vi "GetImage.vi"(8 "error in (no error)":errorcluster, 10 "index (0 = most recent)":i32) -> (0 "error out":errorcluster, 2 "Img":string)   [LabVIEW 2017, in "SystemController.lvclass"]
doc: "---------------------------------------------------------------\nJKI State Machine Objects™\nhttp://jki.net/state-machine-objects/\nCopyright (C) 2005-2015, JKI <info@jki.net>\nALL RIGHTS RESERVEDJKI State Machine Objects (SMO) 1.0.0.5\nJKI - JKI\nCopyright (c) 2016, JKI"
uses:
  SystemController.lvclass
panel:
  # "For instructions on how to use the JKI State Machine Objects, examples and video tutorials, visit:\nhttp://jki.net/state-machine-objects/\n\nJKI State Machine Objects™\nhttp://jki.net/state-machine-objects/\nCopyright (C) 2005-2015, JKI <info@jki.net>\nALL RIGHTS RESERVED"
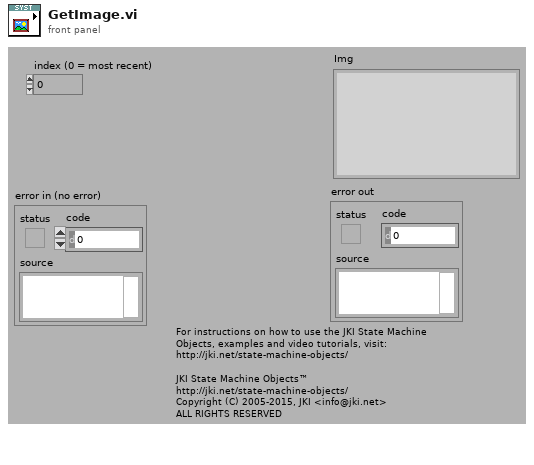
[diagram p1: front panel]
types:
  T1 = typedef "IMAQ Image.ctl" = refnum<image>
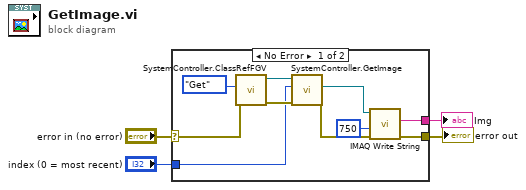
[diagram p0: block diagram]
diagram:
  n1 = case shown="No Error" "error in (no error)" {
    selector: "error in (no error)" -> [w6 w15]
    tunnel: [w9 w15] -> w4
    tunnel: [w7 _] -> w3
    tunnel: "index (0 = most recent)" -> [w5 _]
    frame No Error {
      n2 = call "SystemController.ClassRefFGV.vi"("error in (no error)"=w6, "Set/Get"=enum16{"Set", "Get"}."Get") -> ("error out"=w12:errorcluster, "SystemController out"=w13:refnum<class "SystemController.lvclass">)  [unwired: 8 in]
      n3 = call "SystemController.GetImage.vi"("error in (no error)"=w12, "index (0 = most recent)"=w5, "SystemController"=w13) -> ("error out"=w10:errorcluster, "Image"=w8:T1)  [unwired: 6 in, 1 out]
      n4 = call-poly "IMAQ Write String"("error in (no error)"=w10, "Image Quality"=u32 750, "Image"=w8) -> ("error out"=w9:errorcluster, "FileString"=w7:string)  [unwired: 6 in, 1 out]
    }
    frame Error {
    }
  }
  "Img" <- w3
  "error out" <- w4
